vi "Pick Right.vi"(4 "Threshold":sgl=10.0, 5 "Pause on Miss?":bool, 6 "Target Position":sgl=31.0, 7 "Pick":T1, 8 "error in":errorcluster, 11 "Location":string="Base") -> (0 "error out":errorcluster, 3 "Location Out":string=" ")   [LabVIEW 2013]
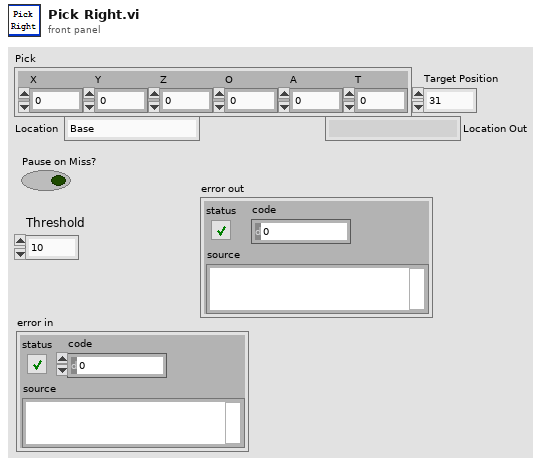
[diagram p1: front panel]
types:
  T1 = cluster{"X":dbl, "Y":dbl, "Z":dbl, "O":dbl, "A":dbl, "T":dbl}
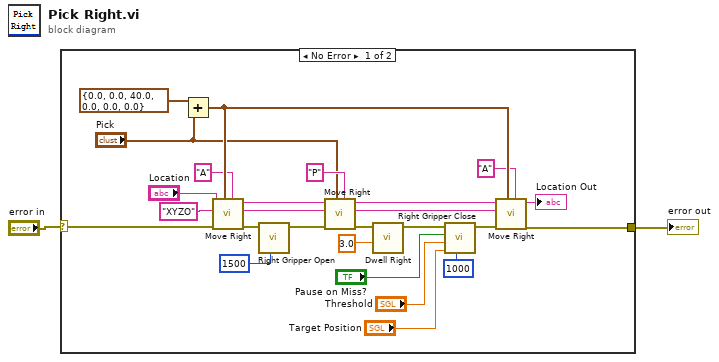
[diagram p0: block diagram]
diagram:
  n1 = case shown="No Error" "error in" {
    selector: "error in" -> [w13 w29]
    tunnel: [w14 w29] -> w2
    frame No Error {
      n2 = Add(x=T1 {"X"=0.0, "Y"=0.0, "Z"=40.0, "O"=0.0, "A"=0.0, "T"=0.0} ("Pick"), y="Pick") -> (x+y=w18:T1)
      n3 = call "Move Right.vi"("Label"="A", "Goal"=w18, "error in"=w13, "Mask"="XYZO", "Location"="Location") -> ("error out"=w26:errorcluster, "Mask Out"=w28:string, "Location Out"=w8:string)  [unwired: 2 in, 2 out]
      n4 = call "Right Gripper Open.vi"("Delay"=u32 1500, "error in"=w26) -> ("error out"=w20:errorcluster)  [unwired: 9 in]
      n5 = call "Move Right.vi"("Label"="P", "Goal"="Pick", "error in"=w20, "Mask"=w28, "Location"=w8) -> ("error out"=w23:errorcluster, "Mask Out"=w27:string, "Location Out"=w7:string)  [unwired: 2 in, 2 out]
      n6 = call "Dwell Right.vi"("Wait Time"=3.0, "error in"=w23) -> ("error out"=w24:errorcluster)  [unwired: 9 in]
      n7 = call "Right Gripper Close.vi"("Delay"=u32 1000, "Target Position"="Target Position", "Threshold"="Threshold", "Pause on Miss?"="Pause on Miss?", "error in"=w24) -> ("error out"=w19:errorcluster)  [unwired: 5 in, 1 out]
      n8 = call "Move Right.vi"("Label"="A", "Goal"=w18, "error in"=w19, "Mask"=w27, "Location"=w7) -> ("error out"=w14:errorcluster, "Location Out"=→"Location Out":string)  [unwired: 2 in, 3 out]
    }
    frame Error {
    }
  }
  "error out" <- w2
